vi "MGI Generate Rotation Matrix.vi"(1 "Rotation Axis":T1, 2 "Right Hand Rotation":dbl format="%.2f") -> (0 "Rotation Matrix[3][3]":dbl[][](array[numeric]) format="%.2f")   [LabVIEW 2016]
doc: "Generate a 3x3 rotation matrix with specified diagonal elements, +/- the off diagonal element, and specified axis unrotated.\n\nAuthored by David A. Moore\nsupport@mooregoodideas.com\nwww.mooregoodideas.com\n\nCopyright (c) 2010, Moore Good Ideas, Inc.\n\nAll rights reserved.\n\nRedistribution and use in source and binary forms, with or without modification, are permitted provided that the following conditions are met:\n\n * Redistributions of source code must retain the above copyright notice, this list of conditions and the following disclaimer.\n * Redistributions in binary form must reproduce the above copyright notice, this list of conditions and the following disclaimer in the documentation and/or other materials provided with the distribution.\n * Neither the name of Moore Good Ideas, Inc. nor the names of its contributors may be used to endorse or promote products derived from this software without specific prior written permission.\n\nTHIS SOFTWARE IS PROVIDED BY THE COPYRIGHT HOLDERS AND CONTRIBUTORS \"AS IS\" AND ANY EXPRESS OR IMPLIED WARRANTIES, INCLUDING, BUT NOT LIMITED TO, THE IMPLIED WARRANTIES OF MERCHANTABILITY AND FITNESS FOR A PARTICULAR PURPOSE ARE DISCLAIMED. IN NO EVENT SHALL THE COPYRIGHT OWNER OR CONTRIBUTORS BE LIABLE FOR ANY DIRECT, INDIRECT, INCIDENTAL, SPECIAL, EXEMPLARY, OR CONSEQUENTIAL DAMAGES (INCLUDING, BUT NOT LIMITED TO, PROCUREMENT OF SUBSTITUTE GOODS OR SERVICES; LOSS OF USE, DATA, OR PROFITS; OR BUSINESS INTERRUPTION) HOWEVER CAUSED AND ON ANY THEORY OF LIABILITY, WHETHER IN CONTRACT, STRICT LIABILITY, OR TORT (INCLUDING NEGLIGENCE OR OTHERWISE) ARISING IN ANY WAY OUT OF THE USE OF THIS SOFTWARE, EVEN IF ADVISED OF THE POSSIBILITY OF SUCH DAMAGE."
uses:
  <userlib>/_MGI/Coordinates/MGI Coordinate Axis Enum.ctl
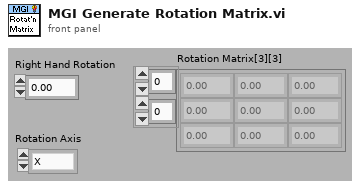
[diagram p1: front panel]
types:
  T1 = typedef "MGI Coordinate Axis Enum.ctl" = enum16{"X", "Y", "Z"}
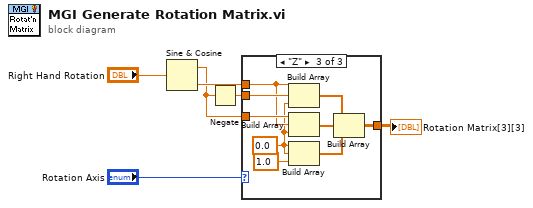
[diagram p0: block diagram]
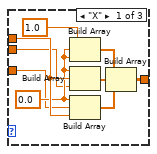
[diagram p2: hidden frame]
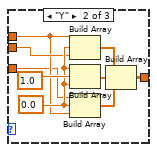
[diagram p3: hidden frame]
diagram:
  n1 = Sine & Cosine(0:"Right Hand Rotation") -> (1:w1:dbl, 2:w4:dbl)
  n2 = Negate(x=w1) -> (-x=w2:dbl)
  n3 = case shown="\"Z\"" "Rotation Axis" {
    tunnel: w2 -> [w9 w18 w30]
    tunnel: w1 -> [w8 w16 w29]
    tunnel: w4 -> [w12 w17 w28]
    tunnel: [w13 w21 w25] -> w5
    frame "X" {
      w11 = 0.0 ("Input Element")
      n4 = Build Array(1.0 ("Input Element"), w11, w11) -> (w15:dbl[])
      n5 = Build Array(w11, w12, w9) -> (w7:dbl[])
      n6 = Build Array(w11, w8, w12) -> (w14:dbl[])
      n7 = Build Array(w15, w7, w14) -> (w13:dbl[][])
    }
    frame "Y" {
      w19 = 0.0 ("Input Element")
      n8 = Build Array(w17, w19, w18) -> (w23:dbl[])
      n9 = Build Array(w19, 1.0 ("Input Element"), w19) -> (w24:dbl[])
      n10 = Build Array(w16, w19, w17) -> (w22:dbl[])
      n11 = Build Array(w23, w24, w22) -> (w21:dbl[][])
    }
    frame "Z" {
      w26 = 0.0 ("Input Element")
      n12 = Build Array(w28, w30, w26) -> (w32:dbl[])
      n13 = Build Array(w29, w28, w26) -> (w33:dbl[])
      n14 = Build Array(w26, w26, 1.0 ("Input Element")) -> (w31:dbl[])
      n15 = Build Array(w32, w33, w31) -> (w25:dbl[][])
    }
  }
  "Rotation Matrix[3][3]" <- w5
